vi "example_cmd.vi"() -> ()   [LabVIEW 2015]
uses:
  dotnet_system_exec/dotnet_system_exec.lvclass
panel:
  in  "working directory":path=path "c:/"
  out "StdErr":string
  out "StdOut":string
  in  "Send":bool
  in  "Cmd In (can include multiple lines)":string="dir"
  in  "Stop":bool
  # "This examples launches the cmd.exe process and allows you to send strings via stdin, while asynchronously listening to stdout and stderr"
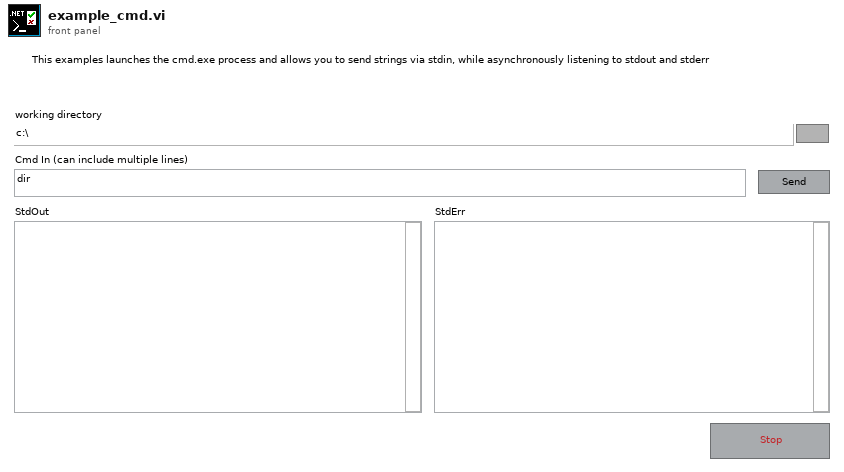
[diagram p1: front panel]
types:
  T1 = cluster{"stdout event":refnum<user-event>, "stdout event":refnum<user-event>}
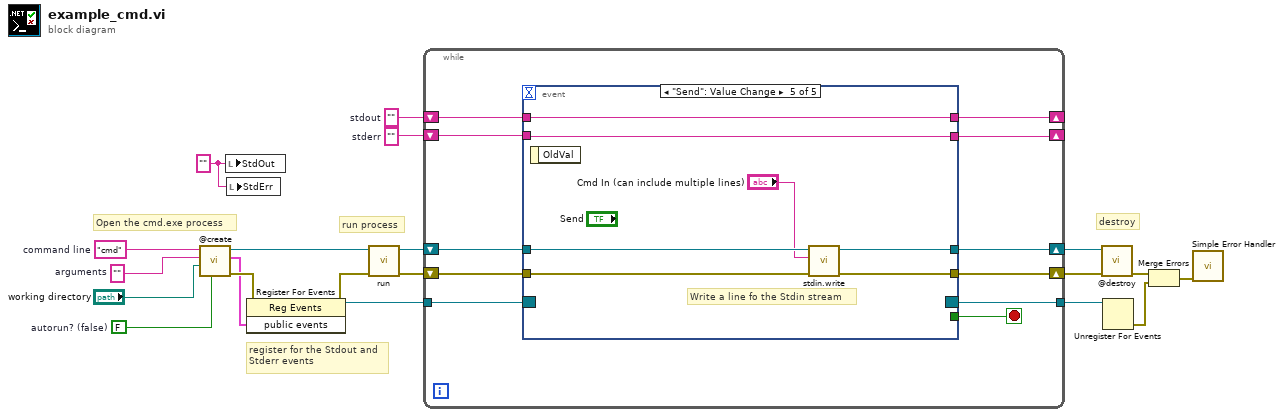
[diagram p0: block diagram]
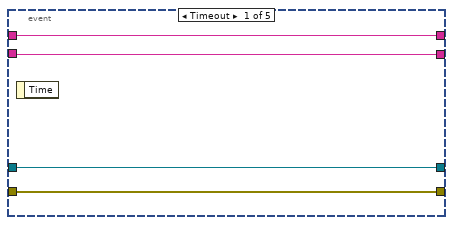
[diagram p2: hidden frame]
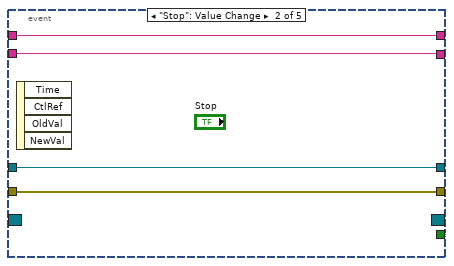
[diagram p3: hidden frame]
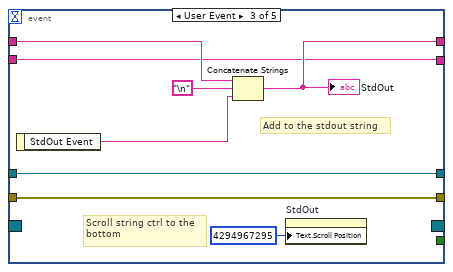
[diagram p4: hidden frame]
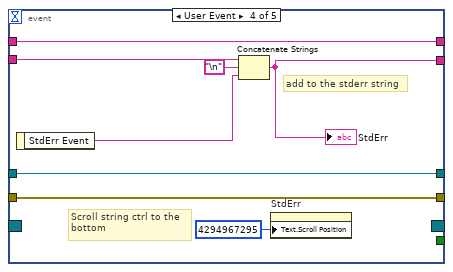
[diagram p5: hidden frame]
diagram:
  w1 = FALSE  # autorun? (false)
  w2 = "" ("Process File Name")
  w4 = ""  # stderr
  w9 = ""  # arguments
  w10 = ""  # stdout
  w11 = "cmd"  # command line
  # "destroy"
  # "register for the Stdout and\nStderr events"
  # "run process"
  # "Open the cmd.exe process"
  n1 = call "@create.vi"("autorun? (false)"=w1, "working directory (\"\")"="working directory", "arguments (\"\")"=w9, "command line (cmd.exe)"=w11) -> ("error out"=w7:errorcluster, "public events"=w5:T1, "dotnet_system_exec out"=w18:refnum<class "dotnet_system_exec.lvclass">)  [unwired: 5 in]
  n2 = local write "StdOut"(w2) -> ()
  n3 = local write "StdErr"(w2) -> ()
  n4 = register-events(error in=w7, w5) -> (reference out=w17:refnum<event-registration>, error out=w6:errorcluster)  [unwired: 1 in]
  n5 = call "run.vi"("error in (no error)"=w6, "dotnet_system_exec in"=w18) -> ("error out"=w8:errorcluster, "dotnet_system_exec out"=w20:refnum<class "dotnet_system_exec.lvclass">)  [unwired: 8 in]
  n6 = while {
    shift-right: [w31] -> w19
    shift-left: w20 -> [w30]
    shift-right: [w28] -> w15
    shift-left: w8 -> [w29]
    tunnel: w17 -> [w27]
    tunnel: [w26] -> w16
    shift-right: [w24] -> _
    shift-left: w10 -> [w25]
    shift-right: [w21] -> _
    shift-left: w4 -> [w22]
    stop <- w23 stop-if-true
    n7 = event shown="[4] \"Send\": Value Change" {
      selector: w27 -> [_ _ _ _ _]
      dyn-events: [_ _ _ _ _] -> w26
      timeout: _ -> [_ _ _ _ _]
      tunnel: [w35 w40 w48 w56 w63] -> w31
      tunnel: w30 -> [w35 w40 w48 w56 w62]
      tunnel: w29 -> [w34 w39 w47 w55 w60]
      tunnel: [w34 w39 w47 w55 w61] -> w28
      tunnel: w25 -> [w33 w37 w44 w51 w58]
      tunnel: [w33 w37 w45 w51 w58] -> w24
      tunnel: [_ TRUE _ _ _] -> w23
      tunnel: w22 -> [w32 w36 w42 w52 w57]
      tunnel: [w32 w36 w42 w50 w57] -> w21
      event Timeout {
        n8 = event-data() -> ()  [unwired: 1 in, 1 out]
      }
      event "Stop": Value Change {
        n9 = event-data() -> ()  [unwired: 1 in, 4 out]
      }
      event User Event {
        # "Scroll string ctrl to the \nbottom"
        # "Add to the stdout string"
        n10 = event-data() -> ("StdOut Event"=w43:string)  [unwired: 1 in]
        n11 = Concatenate Strings(w44, "\n", w43) -> (w45:string)
        "StdOut" <- w45
        n12 = property on="StdOut" class="Str"("Text.Scroll Position"=u32 4294967295) -> ()  [unwired: 2 in, 2 out]
      }
      event User Event {
        # "Scroll string ctrl to the \nbottom"
        # "add to the stderr string"
        n13 = event-data() -> ("StdErr Event"=w53:string)  [unwired: 1 in]
        n14 = Concatenate Strings(w52, "\n", w53) -> (w50:string)
        "StdErr" <- w50
        n15 = property on="StdErr" class="Str"("Text.Scroll Position"=u32 4294967295) -> ()  [unwired: 2 in, 2 out]
      }
      event "Send": Value Change {
        # "Write a line fo the Stdin stream"
        n16 = event-data() -> ()  [unwired: 1 in, 1 out]
        n17 = call-dynamic "stdin.write.vi"("error in (no error)"=w60, "stdin"="Cmd In (can include multiple lines)", "dotnet_system_exec in"=w62) -> ("error out"=w61:errorcluster, "dotnet_system_exec out"=w63:refnum<class "dotnet_system_exec.lvclass">)  [unwired: 7 in]
      }
    }
  }
  n18 = call-dynamic "@destroy.vi"("error in (no error)"=w15, "dotnet_system_exec in"=w19) -> ("error out"=w14:errorcluster)  [unwired: 8 in, 1 out]
  n19 = Unregister For Events(event registration refnum=w16) -> (error out=w13:errorcluster)  [unwired: 1 in]
  n20 = Merge Errors(w14, w13) -> (w12:errorcluster)
  n21 = call <vilib>:"Simple Error Handler.vi"("error in (no error)"=w12) -> ()  [unwired: 4 in, 5 out]
